vi "Intake Get.vi"(1 "Gripper":dbl, 2 "Change arm?":bool) -> (0 "Intake Info Out":T2)   [LabVIEW 2013]
uses:
  <vilib>/Rock Robotics/WPI/Solenoid/WPI_SolenoidValue.ctl
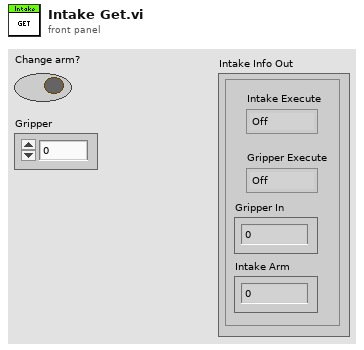
[diagram p1: front panel]
types:
  T1 = typedef "WPI_SolenoidValue.ctl" = enum16{"Off", "On", "Forward", "Reverse"}
  T2 = cluster{"Intake Execute":T1, "Gripper Execute":T1, "Gripper In":dbl, "Intake Arm":dbl}
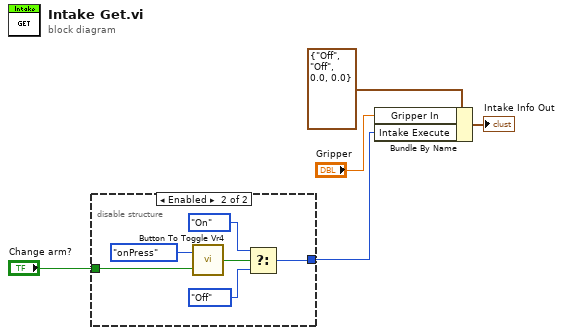
[diagram p0: block diagram]
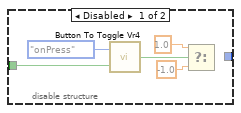
[diagram p2: hidden frame]
diagram:
  n1 = disable-structure shown="Enabled" {
    disable-tunnel: "Change arm?" -> [w10 w12]
    disable-tunnel: [_ w16] -> w2
    frame Disabled {
      n2 = call "Button To Toggle Vr4.vi"("InValue"=w10, "Action"=enum16{"onPress", "onRelease", "Both"}."onPress") -> ("Result"=w8:bool)
      n3 = Select(t=1.0, s=w8, f=-1.0) -> ()  [unwired: 1 out]
    }
    frame Enabled {
      n4 = call "Button To Toggle Vr4.vi"("InValue"=w12, "Action"=enum16{"onPress", "onRelease", "Both"}."onPress") -> ("Result"=w11:bool)
      n5 = Select(t=WPI_SolenoidValue."On" ("Gripper Execute"), s=w11, f=WPI_SolenoidValue."Off" ("Gripper Execute")) -> (s? t:f=w16:T1)
    }
  }
  n6 = Bundle By Name(cluster=T2 {"Intake Execute"=enum."Off", "Gripper Execute"=enum."Off", "Gripper In"=0.0, "Intake Arm"=0.0} ("Intake Info Out"), "Gripper In"="Gripper", "Intake Execute"=w2) -> (→"Intake Info Out":T2)
